vi "GUI Init - DIM3.vi"(7 "Disabled":T1(ring), 8 "error in (no error)":errorcluster, 9 "Ch.names":string[](array[string]), 10 "Cluster":T3, 11 "GUI Refs":T2) -> (0 "error out":errorcluster, 2 "Data":dbl[](array[numeric]), 3 "reference out":refnum<vi>)   [LabVIEW 2017]
doc: "Initialize array's size and values for DIM3 Array by reference"
uses:
  Controls/Discrete_GUI_Cluster.ctl
  Controls/GUI Referencies.ctl
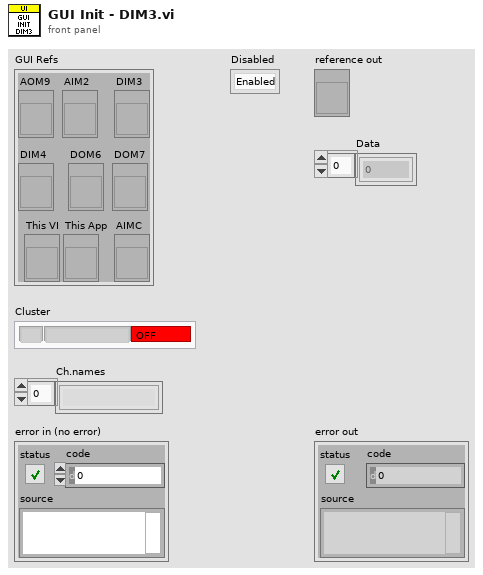
[diagram p1: front panel]
types:
  T1 = enum8{"Enabled", "Disabled", "Disabled and Grayed Out"}
  T2 = typedef "GUI Referencies.ctl" = cluster{"This VI":refnum<vi>, "This App":refnum<vi>, "DIM3":refnum<vi>, "DIM4":refnum<vi>, "DOM6":refnum<vi>, "DOM7":refnum<vi>, "AOM9":refnum<vi>, "AIM2":refnum<vi>, "AIMC":refnum<vi>}
  T3 = typedef "Discrete_GUI_Cluster.ctl" = cluster{"Ch.name":string, "Ch.state":bool, "Num":string}
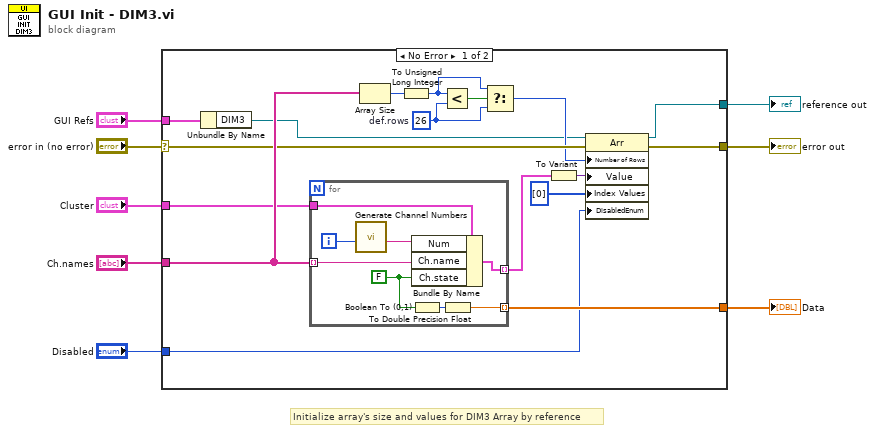
[diagram p0: block diagram]
diagram:
  # "Initialize array's size and values for DIM3 Array by reference"
  n1 = case shown="No Error" "error in (no error)" {
    selector: "error in (no error)" -> [w20 w34]
    tunnel: [w19 w34] -> w7
    tunnel: "Ch.names" -> [w23 _]
    tunnel: "GUI Refs" -> [w22 _]
    tunnel: "Cluster" -> [w21 _]
    tunnel: [w18 _] -> w4
    tunnel: [w10 _] -> w2
    tunnel: "Disabled" -> [w9 _]
    frame No Error {
      w14 = u32 26  # def.rows
      n2 = Unbundle By Name(w22) -> ("DIM3"=w11:refnum<vi>)
      n3 = for {
        tunnel: [w33] -> w17 mode=indexing
        tunnel: w23 -> [w32] mode=indexing
        tunnel: w21 -> [w31]
        tunnel: [w28] -> w18 mode=indexing
        i -> [w26]
        w29 = FALSE
        n4 = call "Generate Channel Numbers.vi"("Index"=w26) -> ("Number"=w27:string)  [unwired: 9 in, 1 out]
        n5 = Bundle By Name(cluster=w31, "Num"=w27, "Ch.name"=w32, "Ch.state"=w29) -> (w33:T3)
        n6 = Boolean To (0,1)(Boolean=w29) -> (0, 1=w30:i16)
        n7 = To Double Precision Float(number=w30) -> (double precision float=w28:dbl)
      }
      n8 = Array Size(array=w23) -> (size(s)=w24:i32)
      n9 = To Unsigned Long Integer(number=w24) -> (unsigned 32bit integer=w13:u32)
      n10 = Less?(x=w13, y=w14) -> (x < y?=w15:bool)
      n11 = Select(t=w13, s=w15, f=w14) -> (s? t:f=w12:u32)
      n12 = To Variant(anything=w17) -> (Variant=w16:variant)
      n13 = property class="Arr"(reference=w11, error in=w20, "Number of Rows"=w12, "Value"=w16, "Index Values"=u32[] [0], "DisabledEnum"=w9) -> (reference out=w10:refnum<vi>, error out=w19:errorcluster)
    }
    frame Error {
    }
  }
  "error out" <- w7
  "Data" <- w4
  "reference out" <- w2
